vi "Write Record(sec).vi"(8 "error in (no error)":errorcluster, 10 "Record":T1, 11 "Configuration Database Actor in":refnum<class "Configuration Database Actor.lvclass">) -> (0 "error out":errorcluster, 3 "Configuration Database Actor out":refnum<class "Configuration Database Actor.lvclass">)   [LabVIEW 2019, in "Configuration Database Actor.lvlib" / "Configuration Database Actor.lvclass"]
uses:
  Configuration Database Actor.lvclass
  Record -Cluster.ctl
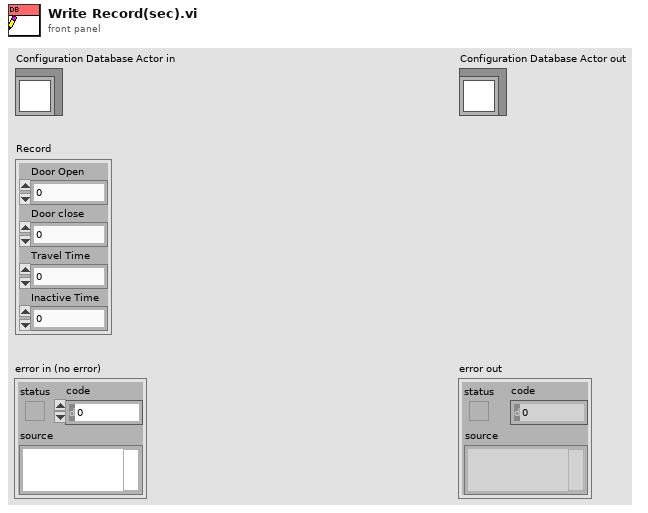
[diagram p1: front panel]
types:
  T1 = typedef "Configuration Database Actor.lvlib/Configuration Database Actor.lvclass/Record -Cluster.ctl" = cluster{"Door Open":dbl, "Door close":dbl, "Travel Time":dbl, "Inactive Time":dbl}
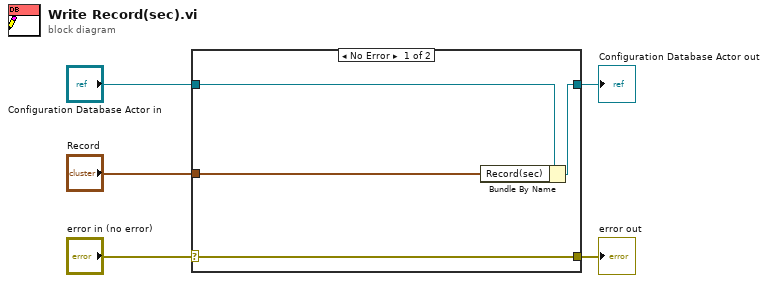
[diagram p0: block diagram]
diagram:
  n1 = case shown="No Error" "error in (no error)" {
    selector: "error in (no error)" -> [w9 w10]
    tunnel: [w9 w10] -> w4
    tunnel: [w7 w11] -> w2
    tunnel: "Configuration Database Actor in" -> [w8 w11]
    tunnel: "Record" -> [w6 _]
    frame No Error {
      n2 = Bundle By Name(cluster=w8, "Record(sec)"=w6) -> (w7:refnum<class "Configuration Database Actor.lvclass">)
    }
    frame Error {
    }
  }
  "error out" <- w4
  "Configuration Database Actor out" <- w2
